vi "sv_Get Component String.vi"(4 "spectrum component":u16(ring)=32 items=["Magnitude^2"=37, "Magnitude"=32, "Phase"=33, "Real"=34, "Imaginary"=35, "Coherence"=36, "Unknown"=99]) -> (1 "x-domain string":string)   [LabVIEW 2017]
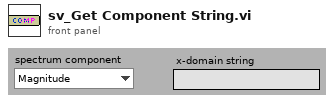
[diagram p1: front panel]
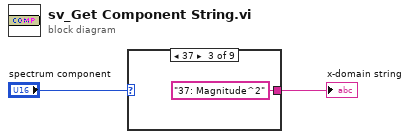
[diagram p0: block diagram]
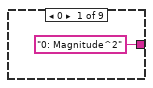
[diagram p2: hidden frame]
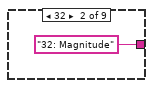
[diagram p3: hidden frame]
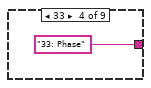
[diagram p4: hidden frame]
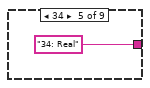
[diagram p5: hidden frame]
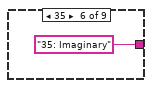
[diagram p6: hidden frame]
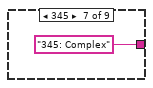
[diagram p7: hidden frame]
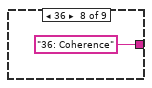
[diagram p8: hidden frame]
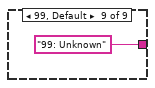
[diagram p9: hidden frame]
diagram:
  n1 = case shown="37" "spectrum component" {
    tunnel: ["0: Magnitude^2" ("t") "32: Magnitude" ("t") "37: Magnitude^2" ("t") "33: Phase" ("t") "34: Real" ("t") "35: Imaginary" ("t") "345: Complex" ("t") "36: Coherence" ("t") "99: Unknown" ("t")] -> w1
    frame 0 {
    }
    frame 32 {
    }
    frame 37 {
    }
    frame 33 {
    }
    frame 34 {
    }
    frame 35 {
    }
    frame 345 {
    }
    frame 36 {
    }
    frame 99, Default {
    }
  }
  "x-domain string" <- w1
